vi "set_multiramp_soak_profile_configuration.vi"(6 "Tracking enabled":bool, 8 "error in (no error)":errorcluster, 9 "Segment number":u8 max=15, 10 "Program number":u8 max=99, 11 "connection ID":refnum<k5>) -> (0 "error out":errorcluster, 3 "connection ID out":refnum<k5>)   [LabVIEW 2018]
panel:
  out "bytes written":i32
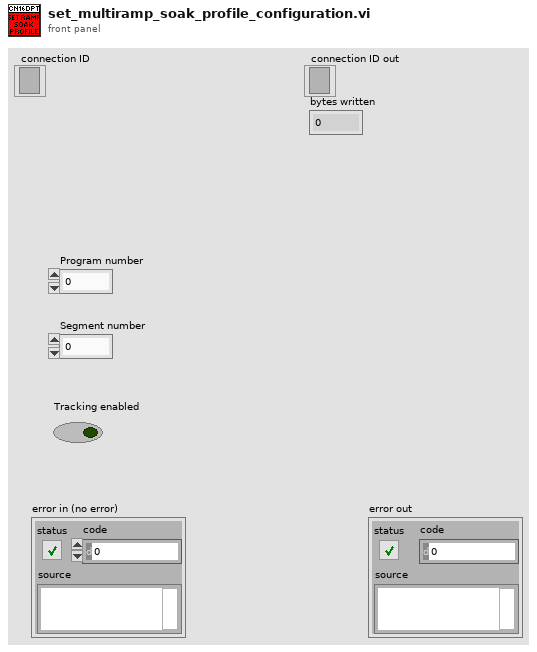
[diagram p1: front panel]
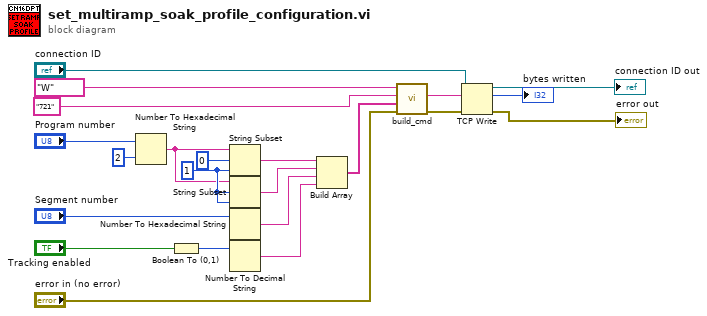
[diagram p0: block diagram]
diagram:
  w8 = 1 ("length (rest)")
  n1 = Number To Hexadecimal String(1:i16 2 ("width (-)"), 2:"Program number") -> (0:w7:string)
  n2 = Boolean To (0,1)(Boolean="Tracking enabled") -> (0, 1=w14:i16)
  n3 = String Subset(string=w7, offset (0)=0, length (rest)=w8) -> (substring=w6:string)
  n4 = String Subset(string=w7, offset (0)=w8, length (rest)=w8) -> (substring=w5:string)
  n5 = Number To Hexadecimal String(2:"Segment number") -> (0:w4:string)  [unwired: 1 in]
  n6 = Number To Decimal String(number=w14) -> (decimal integer string=w13:string)  [unwired: 1 in]
  n7 = Build Array(w6, w5, w4, w13) -> (w16:string[])
  n8 = call "build_cmd.vi"("error in (no error)"="error in (no error)", "Parameter list"=w16, "Command ID"="721", "Command class"="W") -> ("error out"=w19:errorcluster, "Command"=w18:string)  [unwired: 6 in]
  n9 = TCP Write(connection ID="connection ID", data in=w18, error in (no error)=w19) -> (connection ID out=→"connection ID out":refnum<k5>, bytes written=→"bytes written":i32, error out=→"error out":errorcluster)  [unwired: 1 in]
